vi "lorentzian from circle corners - i.vi"(6 "fragment  : cursor window":T4={"left"=2378.60310421286, "right "=2421.6740576496672, "center"=2421.6740576496672, "window"=2421.6740576496672, "cursors"=[], "relative"=0, "absolute"=0, "fixed vertical offset"=2421.6740576496672, "vertical offset"=2421.6740576496672, "skew"=2421.6740576496672, "default window frac"=2421.6740576496672, "kind"=enum."symmetric", "skew.left"=2421.6740576496672, "skew.right"=2421.6740576496672, "Plot ref"=refnum, "wing order"=enum."back"}, 7 "update z(inf)":enum16{"update z(inf)", "do not update z(inf)"}(ring)=enum."do not update z(inf)", 8 "omega map rameters in":T5={"map method"=enum."less trivial", "2:window factor"=1, "left"=3.0, "right"=3.0, "omega"=3.0, "gamma"=3.0, "theta0"=3.0, "use points"=enum."decimated", "z(inf) method"=enum."median"}, 9 "main VI  path":path, 10 "parameters in: center detection":T3={"number of 2D grid points"=200, "# of points in pond"=93, "# of points in window"=4107, "decimation threshold"=1, "normalization factor"=0.005102552585135461, "pond scale factor "=3.0, "normalized z"=[], "decimated z"=[], "decimated omega"=[], "omega in window"=[], "z in window"=[], "data center"=-0.0014901433980738042-0.0014987103874714112i, "inverse"=[], "linear "=[], "omega around"=[], "phase around center"=[], "fit for phase around senter "=[], "three points"={[], []}, "max omega"=0.029014793, "min omega"=0.029014793, "dz/domega"=[]}, 11 "lorentzian in":T1={"Amplitude"=-1.0311345636926572, "omega(0)"=-1.0311345636926572, "Gamma"=-1.0311345636926572, "phase"=-1.0311345636926572, "Q"=-1.0311345636926572, "Norm  Ampl"=-1.0311345636926572, "z (inf)"=-1.0311345636926572+0.0i, "4corners"={"z (-pi/2)"=-1.0311345636926572+0.5736824521422934i, "z(inf)"=-0.5200164984937075+1.0975277942502903i, "z (pi/2)"=-1.0311345636926572+0.5736824521422934i, "z center"=-0.5136528600391839+0.580046090596817i, "z(0)"=-0.5200164984937075+1.0975277942502903i, "radius"=-1.0311345636926572}} {"z (inf)" format="%#9_9f"; "Q" format="%#9_9f"; "phase" format="%#9_9f"; "Gamma" format="%#9_9f"; "omega(0)" format="%#9_9f"}) -> (0 "omega map parameters  out":T5={"map method"=enum."less trivial", "2:window factor"=1, "left"=3.0, "right"=3.0, "omega"=3.0, "gamma"=3.0, "theta0"=3.0, "use points"=enum."decimated", "z(inf) method"=enum."median"}, 2 "parameters out  : center detection":T3={"number of 2D grid points"=200, "# of points in pond"=93, "# of points in window"=4107, "decimation threshold"=1, "normalization factor"=0.005102552585135461, "pond scale factor "=3.0, "normalized z"=[], "decimated z"=[], "decimated omega"=[], "omega in window"=[], "z in window"=[], "data center"=-0.0014901433980738042-0.0014987103874714112i, "inverse"=[], "linear "=[], "omega around"=[], "phase around center"=[], "fit for phase around senter "=[], "three points"={[], []}, "max omega"=0.029014793, "min omega"=0.029014793, "dz/domega"=[]}, 3 "lorentzian out":T1={"Amplitude"=-1.0311345636926572, "omega(0)"=-1.0311345636926572, "Gamma"=-1.0311345636926572, "phase"=-1.0311345636926572, "Q"=-1.0311345636926572, "Norm  Ampl"=-1.0311345636926572, "z (inf)"=-1.0311345636926572+0.0i, "4corners"={"z (-pi/2)"=-1.0311345636926572+0.5736824521422934i, "z(inf)"=-0.5200164984937075+1.0975277942502903i, "z (pi/2)"=-1.0311345636926572+0.5736824521422934i, "z center"=-0.5136528600391839+0.580046090596817i, "z(0)"=-0.5200164984937075+1.0975277942502903i, "radius"=-1.0311345636926572}} {"z (inf)" format="%#9_9f"; "Q" format="%#9_9f"; "phase" format="%#9_9f"; "Gamma" format="%#9_9f"; "omega(0)" format="%#9_9f"})   [LabVIEW 2017]
uses:
  lorentzian.ctl
  circle corners.ctl
  omega map parameters.ctl
  single fit parameters.ctl
  cursor winow.ctl
  <vilib>/Analysis/6fits.llb/Curve Fitting Criteria.ctl
  <vilib>/Utility/error.llb/Clear Errors.vi
  <vilib>/Analysis/baseanly.llb/Median.vi
  <vilib>/Analysis/baseanly.llb/Mean.vi
  <vilib>/Analysis/baseanly.llb/Mean (DBL).vi
  <vilib>/Analysis/2dsp.llb/Unwrap Phase.vi
  <vilib>/gmath/NumericalOptimization/Nonlinear Curve Fit.vi
  <vilib>/gmath/NumericalOptimization/Nonlinear Curve Fit LM.vi
  <vilib>/gmath/interp.llb/Interpolate 1D.vi
  <vilib>/Analysis/NI_AALPro.lvlib
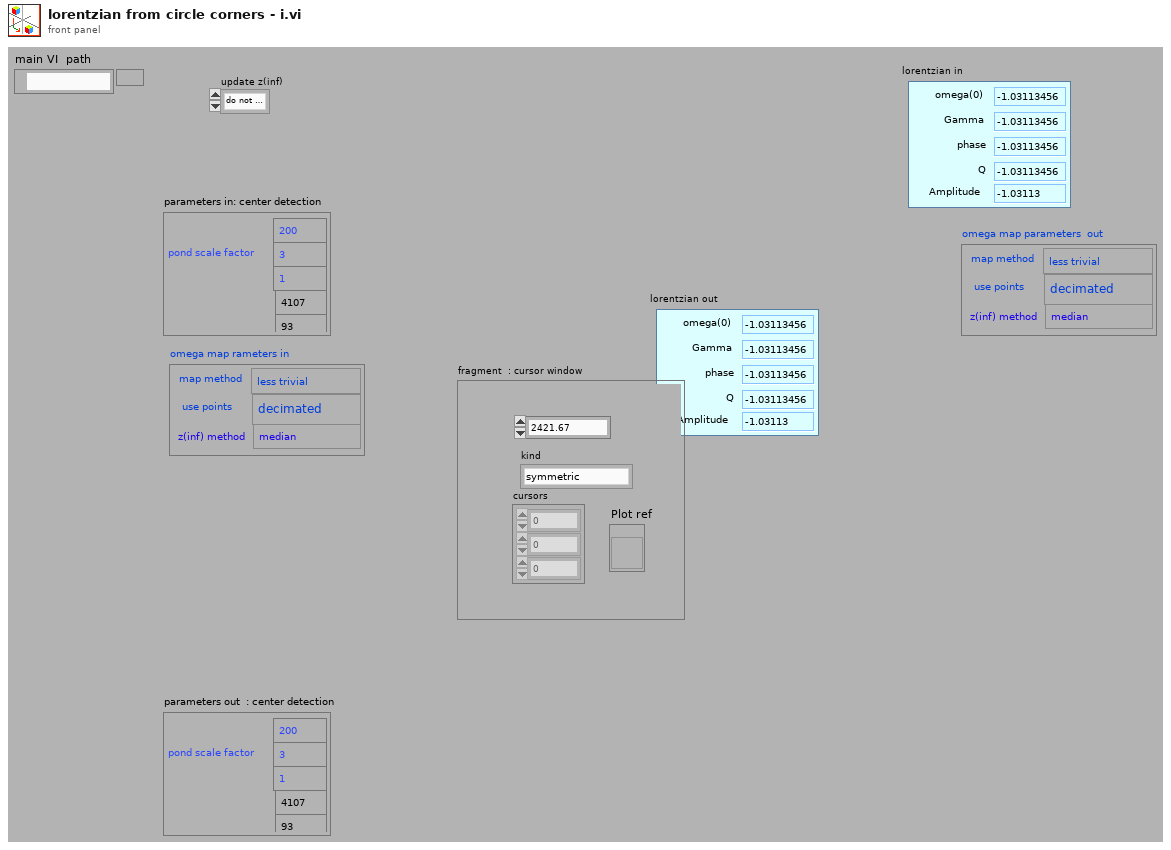
[diagram p1: front panel]
types:
  T1 = typedef "lorentzian.ctl" = cluster{"Amplitude":dbl, "omega(0)":dbl, "Gamma":dbl, "phase":dbl, "Q":dbl, "Norm  Ampl":dbl, "z (inf)":cdb, "4corners":T2}
  T2 = typedef "circle corners.ctl" = cluster{"z (-pi/2)":cdb, "z(inf)":cdb, "z (pi/2)":cdb, "z center":cdb, "z(0)":cdb, "radius":dbl}
  T3 = typedef "single fit parameters.ctl" = cluster{"number of 2D grid points":i32, "# of points in pond":i32, "# of points in window":i32, "decimation threshold":i32, "normalization factor":dbl, "pond scale factor ":dbl, "normalized z":cdb[], "decimated z":cdb[], "decimated omega":dbl[], "omega in window":dbl[], "z in window":cdb[], "data center":cdb, "inverse":cdb[], "linear ":cdb[], "omega around":dbl[], "phase around center":dbl[], "fit for phase around senter ":dbl[], "three points":cluster{dbl[], dbl[]}, "max omega":dbl, "min omega":dbl, "dz/domega":cdb[]}
  T4 = typedef "cursor winow.ctl" = cluster{"left":dbl, "right ":dbl, "center":dbl, "window":dbl, "cursors":i32[], "relative":i32, "absolute":i32, "fixed vertical offset":dbl, "vertical offset":dbl, "skew":dbl, "default window frac":dbl, "kind":enum16{"symmetric", "skewed", "fancy"}, "skew.left":dbl, "skew.right":dbl, "Plot ref":refnum<vi>, "wing order":enum16{"forw", "back"}}
  T5 = typedef "omega map parameters.ctl" = cluster{"map method":enum16{"simple", "less trivial", "around center", "geometry"}, "2:window factor":i32, "left":dbl, "right":dbl, "omega":dbl, "gamma":dbl, "theta0":dbl, "use points":enum16{"all in window", "decimated"}, "z(inf) method":enum16{"median", "method 2", "histogram"}}
  T6 = enum16{"simple", "less trivial", "around center", "geometry"}
  T7 = typedef "NI_AALPro.lvlib/Curve Fitting Criteria.ctl" = u16
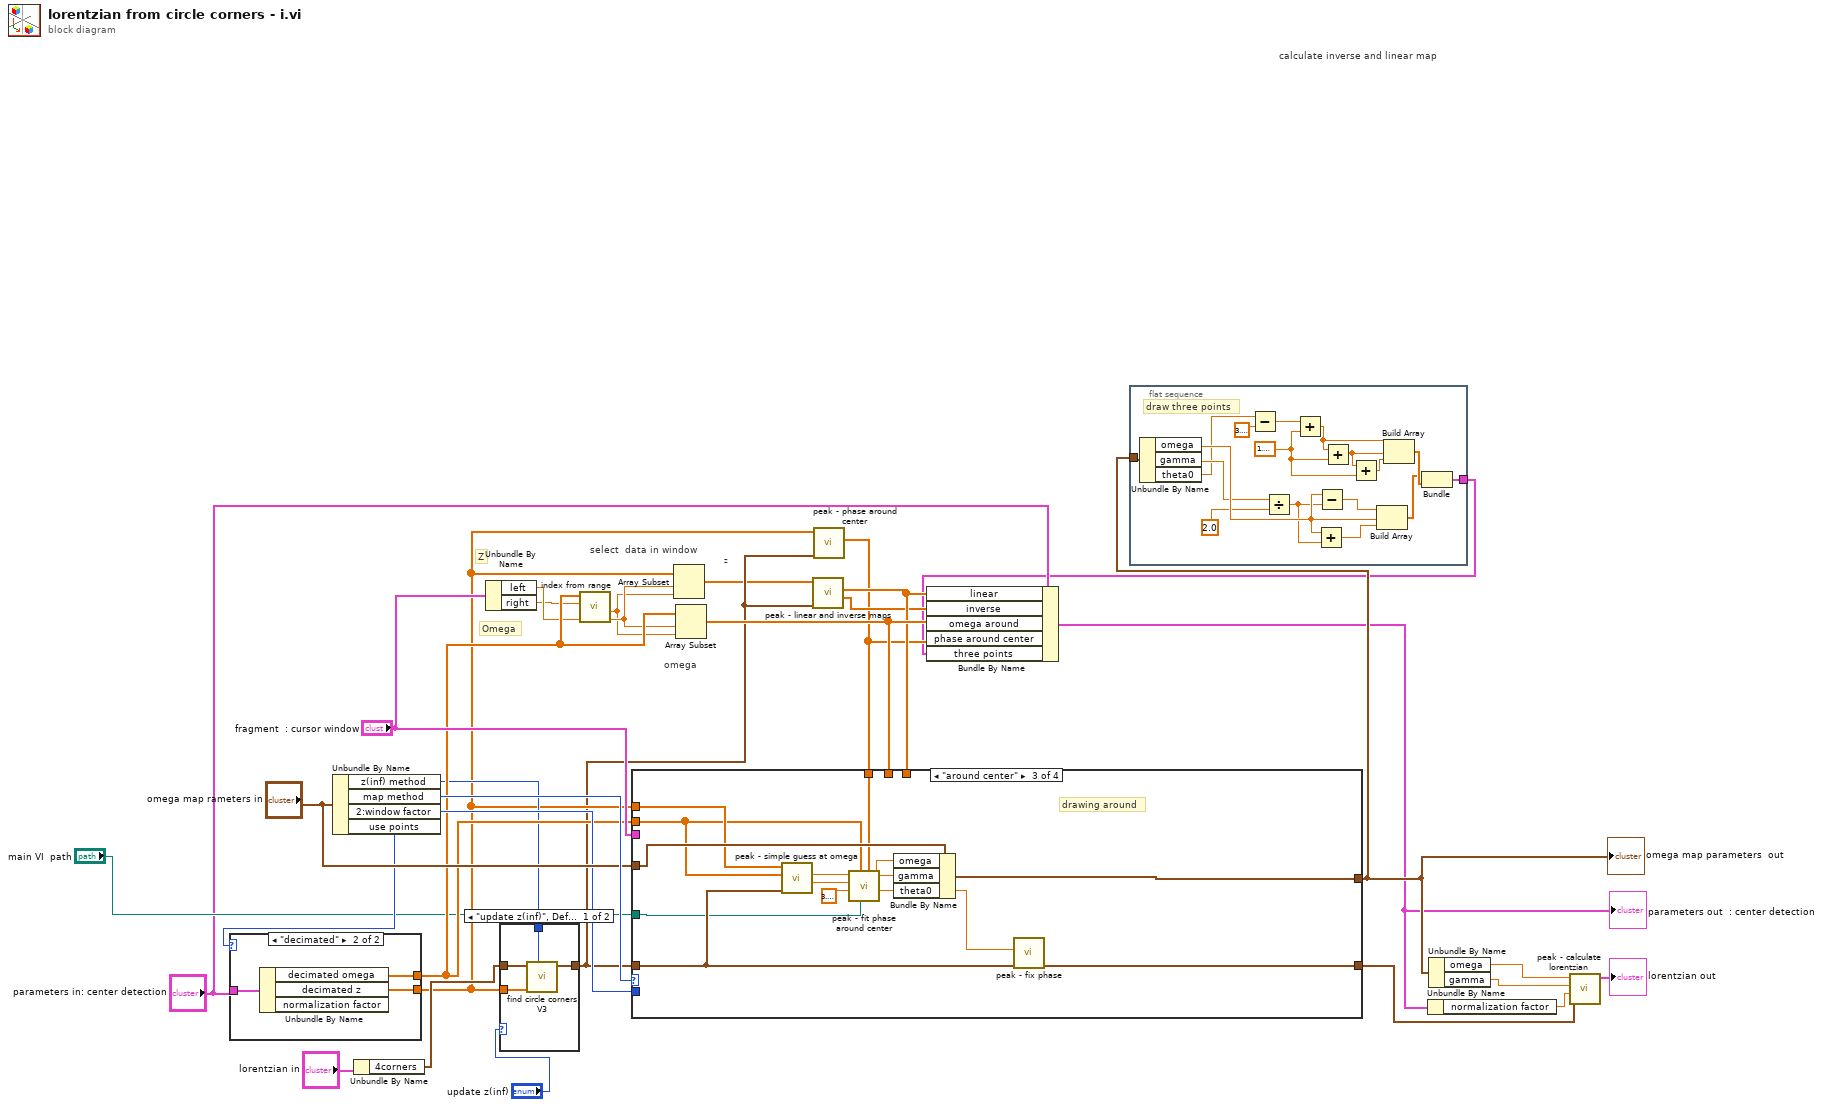
[diagram p0: block diagram]
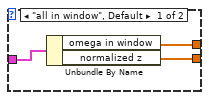
[diagram p3: hidden frame]
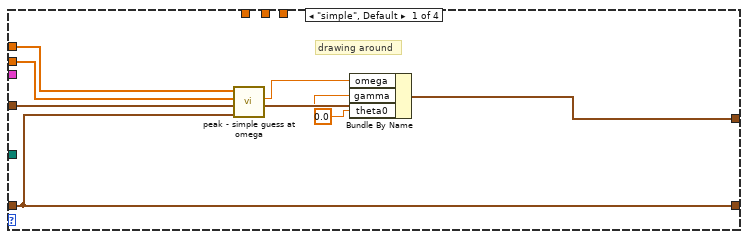
[diagram p4: hidden frame]
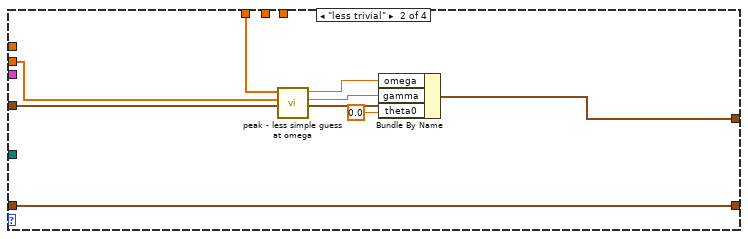
[diagram p5: hidden frame]
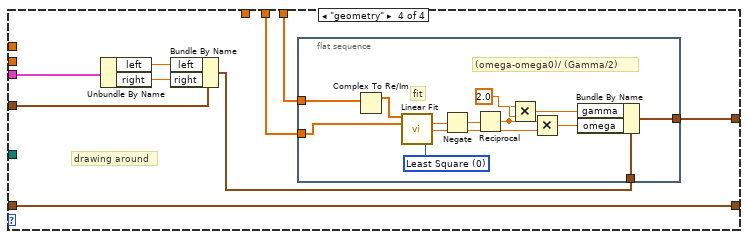
[diagram p6: hidden frame]
diagram:
  # "select  data in window"
  # "omega"
  # "z"
  # "Z"
  # "Omega"
  # "calculate inverse and linear map"
  n1 = Unbundle By Name("omega map rameters in") -> ("z(inf) method"=w20:enum16{"median", "method 2", "histogram"}, "map method"=w31:T6, "2:window factor"=w29:i32, "use points"=w28:enum16{"all in window", "decimated"})
  n2 = case shown="\"decimated\"" w28 {
    tunnel: "parameters in: center detection" -> [w34 w37]
    tunnel: [w33 w36] -> w22
    tunnel: [w32 w35] -> w16
    frame "all in window", Default {
      n3 = Unbundle By Name(w34) -> ("omega in window"=w33:dbl[], "normalized z"=w32:cdb[])
    }
    frame "decimated" {
      n4 = Unbundle By Name(w37) -> ("decimated omega"=w36:dbl[], "decimated z"=w35:cdb[])  [unwired: 1 out]
    }
  }
  n5 = Unbundle By Name("lorentzian in") -> ("4corners"=w19:T2)
  n6 = Unbundle By Name("fragment  : cursor window") -> ("left"=w12:dbl, "right"=w11:dbl)
  n7 = case shown="\"update z(inf)\", Default" "update z(inf)" {
    tunnel: [w40 w42] -> w15
    tunnel: w19 -> [w41 w42]
    tunnel: w16 -> [w39 _]
    tunnel: w20 -> [w38 _]
    frame "update z(inf)", Default {
      n8 = call "find circle corners V3.vi"("method"=w38, "z"=w39, "circle corners in"=w41) -> ("circle corners out"=w40:T2)  [unwired: 8 in]
    }
    frame "do not update z(inf)" {
    }
  }
  n9 = call "index from range.vi"("left"=w12, "right"=w11, "omega"=w22) -> ("left index"=w10:dbl, "length"=w9:dbl)  [unwired: 6 in, 1 out]
  n10 = Array Subset(array=w16, index=w10, length=w9) -> (w14:cdb[])
  n11 = Array Subset(array=w22, index=w10, length=w9) -> (w26:dbl[])
  n12 = call "peak - linear and inverse maps.vi"("4corners"=w15, "Z"=w14) -> ("inverse"=w13:cdb[], "linear"=w24:cdb[])  [unwired: 8 in]
  n13 = call "peak - phase around center.vi"("4corners"=w15, "z"=w16) -> ("Unwrapped Phase"=w3:dbl[])  [unwired: 9 in]
  n14 = case shown="\"around center\"" w31 {
    tunnel: w15 -> [w47 w56 w69 w74]
    tunnel: w16 -> [w46 _ w70 _]
    tunnel: w22 -> [w45 w53 w61 _]
    tunnel: "omega map rameters in" -> [w49 w58 w71 w80]
    tunnel: [w48 w57 w72 w81] -> w5
    tunnel: w29 -> [_ _ _ _]
    tunnel: "fragment  : cursor window" -> [_ _ _ w77]
    tunnel: w26 -> [_ _ _ w76]
    tunnel: w24 -> [_ _ _ w75]
    tunnel: w3 -> [_ w54 w60 _]
    tunnel: [w47 w56 w68 w74] -> w21
    tunnel: "main VI  path" -> [_ _ w59 _]
    frame "simple", Default {
      # "drawing around"
      n15 = call "peak - simple guess at omega.vi"("4corners"=w47, "omega"=w45, "z"=w46) -> ("guess at gamma"=w43:dbl, "guess at omega"=w44:dbl)  [unwired: 7 in]
      n16 = Bundle By Name(cluster=w49, "omega"=w44, "gamma"=w43, "theta0"=0.0 ("phi0")) -> (w48:T5)
    }
    frame "less trivial" {
      n17 = call "peak - less simple guess at omega.vi"("omega"=w53, "Unwrapped Phase"=w54) -> ("gamma guess"=w52:dbl, "omega guess"=w51:dbl)  [unwired: 8 in]
      n18 = Bundle By Name(cluster=w58, "omega"=w51, "gamma"=w52, "theta0"=0.0 ("phi0")) -> (w57:T5)
    }
    frame "around center" {
      # "drawing around"
      n19 = call "peak - simple guess at omega.vi"("4corners"=w69, "omega"=w61, "z"=w70) -> ("guess at gamma"=w66:dbl, "guess at omega"=w67:dbl)  [unwired: 7 in]
      n20 = call "peak - fit phase around center.vi"("Phase"=w60, "main VI  path"=w59, "omega"=w61, "guess at theta"=3.141592653589793, "guess at gamma"=w66, "guess at omega"=w67) -> ("fit for theta"=w62:dbl, "fit for gamma"=w63:dbl, "fit for omega"=w64:dbl)  [unwired: 3 in]
      n21 = Bundle By Name(cluster=w71, "omega"=w64, "gamma"=w63, "theta0"=w62) -> (w72:T5)
      n22 = call "peak - fix phase.vi"("4corners"=w69, "correct phase"=w62) -> ("4corners out"=w68:T2)  [unwired: 9 in]
    }
    frame "geometry" {
      # "drawing around"
      n23 = Unbundle By Name(w77) -> ("left"=w79:dbl, "right"=w78:dbl)
      n24 = Bundle By Name(cluster=w80, "left"=w79, "right"=w78) -> (w73:T5)
      n25 = flat-sequence {
        tunnel: [w94] -> w81
        tunnel: w73 -> [w85]
        tunnel: w76 -> [w84]
        tunnel: w75 -> [w83]
        frame #0 {
          w93 = T7 0 items=["Least Square", "Least Absolute Residual", "Bisquare"] ("method")
          # "(omega-omega0)/ (Gamma/2)"
          # "fit"
          n26 = Complex To Re/Im(x + iy=w83) -> (x=w82:dbl[])  [unwired: 1 out]
          n27 = call <vilib>:"Linear Fit.vi"("Y"=w82, "X"=w84, "method"=w93) -> ("slope"=w91:dbl, "intercept"=w89:dbl)  [unwired: 8 in, 3 out]
          n28 = Negate(x=w91) -> (-x=w90:dbl)
          n29 = Reciprocal(x=w90) -> (1/x=w88:dbl)
          n30 = Multiply(x=w88, y=2.0) -> (x*y=w87:dbl)
          n31 = Multiply(x=w88, y=w89) -> (x*y=w86:dbl)
          n32 = Bundle By Name(cluster=w85, "gamma"=w87, "omega"=w86) -> (w94:T5)
        }
      }
    }
  }
  "omega map parameters  out" <- w5
  n33 = Bundle By Name(cluster="parameters in: center detection", "linear"=w24, "inverse"=w13, "omega around"=w26, "phase around center"=w3, "three points"=w2) -> (w1:T3)
  "parameters out  : center detection" <- w1
  n34 = flat-sequence {
    tunnel: w5 -> [w111]
    tunnel: [w107] -> w2
    frame #0 {
      w99 = 1.5707963267948966
      # "draw three points"
      n35 = Unbundle By Name(w111) -> ("omega"=w110:dbl, "gamma"=w109:dbl, "theta0"=w108:dbl)
      n36 = Subtract(x=w108, y=3.141592653589793) -> (x-y=w95:dbl)
      n37 = Divide(x=w109, y=2.0) -> (x/y=w97:dbl)
      n38 = Add(x=w95, y=w99) -> (x+y=w100:dbl)
      n39 = Add(x=w110, y=w97) -> (x+y=w101:dbl)
      n40 = Subtract(x=w110, y=w97) -> (x-y=w102:dbl)
      n41 = Add(x=w100, y=w99) -> (x+y=w106:dbl)
      n42 = Add(x=w106, y=w99) -> (x+y=w105:dbl)
      n43 = Build Array(w102, w110, w101) -> (w103:dbl[])
      n44 = Build Array(w100, w106, w105) -> (w104:dbl[])
      n45 = Bundle(w103, w104) -> (w107:cluster{dbl[], dbl[]})  [unwired: 1 in]
    }
  }
  n46 = Unbundle By Name(w1) -> ("normalization factor"=w8:dbl)
  n47 = Unbundle By Name(w5) -> ("omega"=w7:dbl, "gamma"=w6:dbl)
  n48 = call "peak - calculate lorentzian.vi"("4corners"=w21, "normalization factor"=w8, "gamma"=w6, "omega"=w7) -> ("lorentzian out"=→"lorentzian out":T1)  [unwired: 7 in]
